vi "niRFUtil CONV dBm to 1 Ohm Voltage (real array).vi"(7 "Real Array (dBm)":T1 min=0 max=127 format="%.2f") -> (8 "Real Array (V)":T1 min=0 max=127 format="%.2f")   [LabVIEW 2015, in "niRFUtil.lvlib"]
doc: "(c) Copyright 2006, National Instruments, Inc. This VI may not be duplicated, sold, or distributed without written consent from National Instruments."
uses:
  niRFUtil.lvlib
  Includes/niRFUtil INC Real Array.ctl
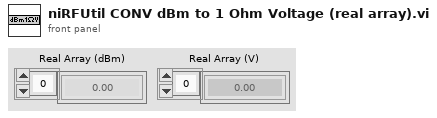
[diagram p1: front panel]
types:
  T1 = typedef "niRFUtil.lvlib/niRFUtil INC Real Array.ctl" = sgl[]
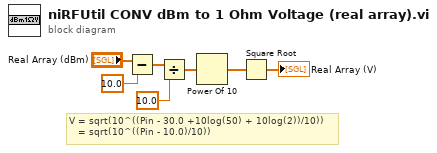
[diagram p0: block diagram]
diagram:
  # "V = sqrt(10^((Pin - 30.0 +10log(50) + 10log(2))/10))\n   = sqrt(10^((Pin - 10.0)/10))"
  n1 = Subtract(x="Real Array (dBm)", y=sgl 10.0) -> (x-y=w6:T1)
  n2 = Divide(x=w6, y=sgl 10.0) -> (x/y=w4:T1)
  n3 = Power Of 10(x=w4) -> (10^x=w3:T1)
  n4 = Square Root(x=w3) -> (sqrt(x)=→"Real Array (V)":T1)
